vi "Expedite the Valley.vi"(0 "Valley in":T2[][](array[typedef]), 1 "Elf Locations in":set{T1}(c389)) -> (2 "Elf Locations out":set{T1}(c389), 3 "Valley out":T2[][](array[typedef]))   [LabVIEW 2020, in "AoC 2022.lvlib"]
uses:
  AoC 2022.lvlib
  Valley Point.ctl
  Valley Item.ctl
  Day 15 - Beacon Exclusion Zone/private/Location.ctl
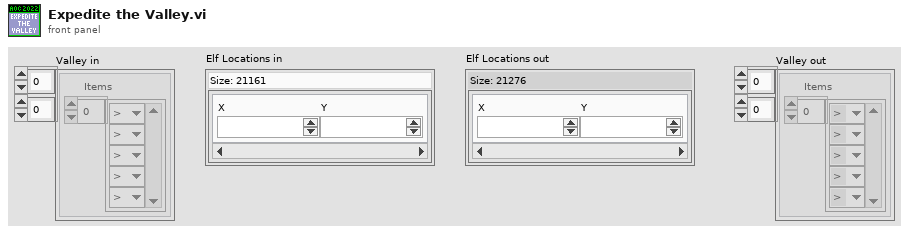
[diagram p1: front panel]
types:
  T1 = typedef "AoC 2022.lvlib/Location.ctl" = cluster{"X":i32, "Y":i32}
  T2 = typedef "AoC 2022.lvlib/Valley Point.ctl" = cluster{"Items":T3[]}
  T3 = typedef "AoC 2022.lvlib/Valley Item.ctl" = enum16{"#", ".", ">", "<", "^", "v", "E"}
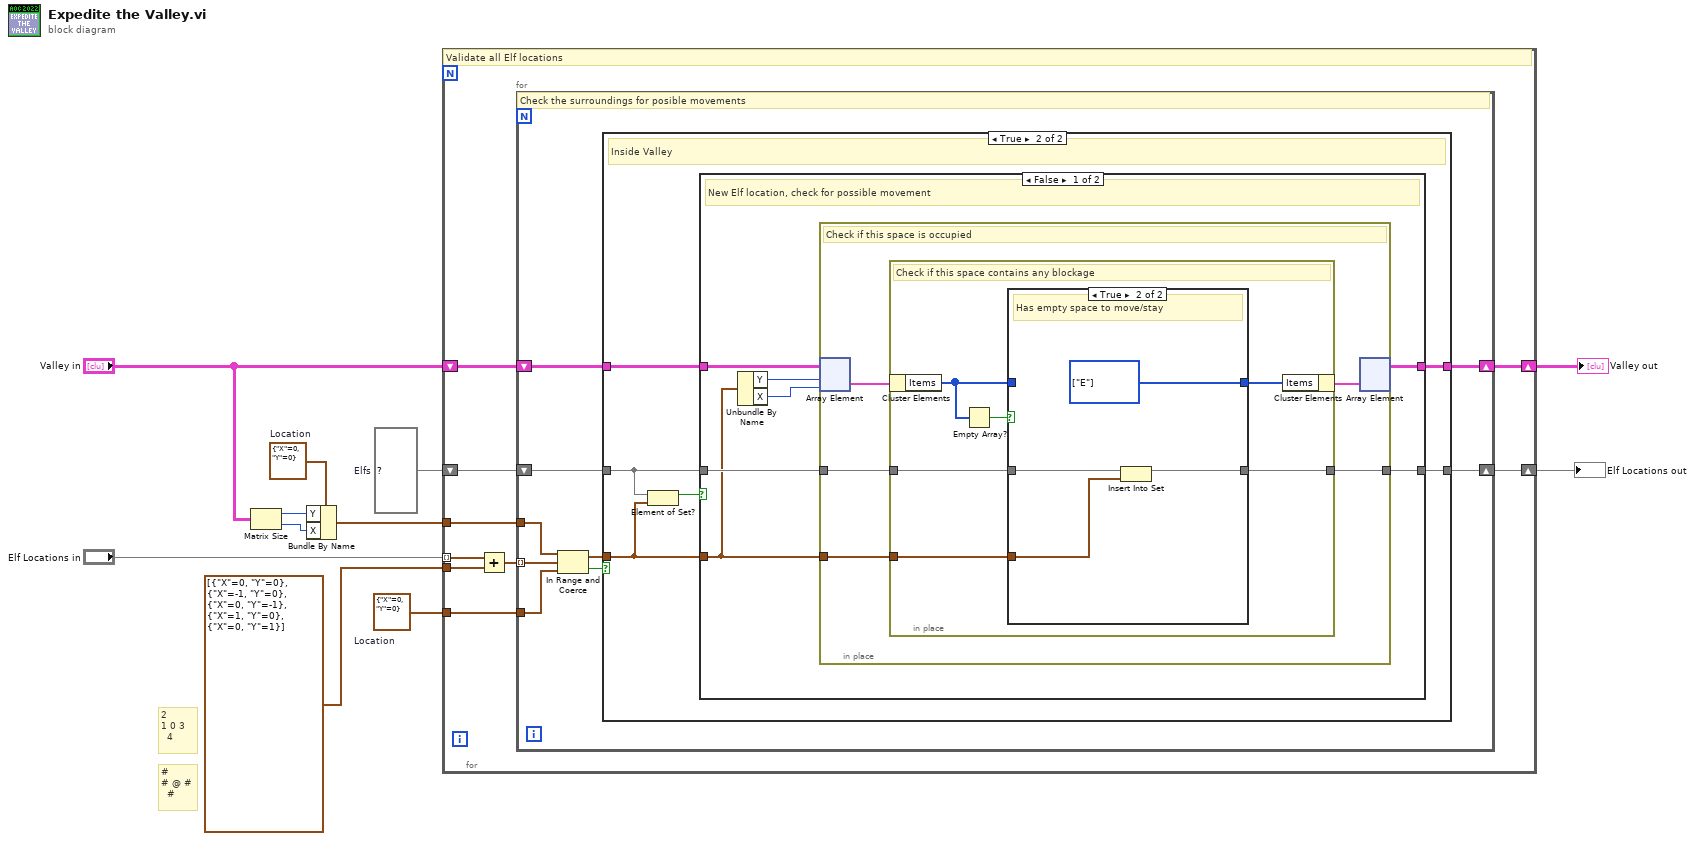
[diagram p0: block diagram]
diagram:
  w2 = set{T1} {}  # Elfs
  w3 = T1 {"X"=0, "Y"=0}  # Location
  w5 = T1 {"X"=0, "Y"=0}  # Location
  # "2  \n1 0 3\n  4"
  # "#  \n# @ #\n  #"
  n1 = Matrix Size(0:"Valley in") -> (1:w7:i32, 2:w6:i32)
  n2 = Bundle By Name(cluster=w5, "Y"=w7, "X"=w6) -> (w8:T1)
  n3 = for {
    shift-right: [w19] -> w11
    shift-left: "Valley in" -> [w20]
    tunnel: T1[] [{"X"=0, "Y"=0}, {"X"=-1, "Y"=0}, {"X"=0, "Y"=-1}, {"X"=1, "Y"=0}, {"X"=0, "Y"=1}] -> [w18]
    tunnel: w8 -> [w17]
    tunnel: "Elf Locations in" -> [w16] mode=indexing
    tunnel: w3 -> [w15]
    shift-right: [w12] -> w1
    shift-left: w2 -> [w13]
    # "Validate all Elf locations"
    n4 = Add(x=w16, y=w18) -> (x+y=w14:T1[])
    n5 = for {
      tunnel: w17 -> [w25]
      tunnel: w14 -> [w27] mode=indexing
      shift-right: [w28] -> w19
      shift-left: w20 -> [w29]
      tunnel: w15 -> [w26]
      shift-right: [w21] -> w12
      shift-left: w13 -> [w22]
      # "Check the surroundings for posible movements"
      n6 = In Range and Coerce(upper limit=w25, x=w27, lower limit=w26) -> (coerced(x)=w23:T1, In Range?=w24:bool)
      n7 = case shown="True" w24 {
        tunnel: w29 -> [w31 w37]
        tunnel: [w31 w36] -> w28
        tunnel: w23 -> [_ w33]
        tunnel: w22 -> [w30 w34]
        tunnel: [w30 w35] -> w21
        frame False {
          # "Outside Valley"
        }
        frame True {
          # "Inside Valley"
          n8 = Element of Set?(10:w33, 11:w34) -> (3:w32:bool)
          n9 = case shown="False" w32 {
            tunnel: w37 -> [w44 w63]
            tunnel: [w43 w63] -> w36
            tunnel: [w40 w62] -> w35
            tunnel: w34 -> [w39 w62]
            tunnel: w33 -> [w38 _]
            frame False {
              # "New Elf location, check for possible movement"
              n10 = Unbundle By Name(w38) -> ("Y"=w42:i32, "X"=w41:i32)
              n11 = in-place {
                in-place-border: w39 -> [w47]
                in-place-border: [w46] -> w40
                in-place-border: w38 -> [w45]
                # "Check if this space is occupied"
                n12 = in-place-array #1(w44, w42, w41) -> (w49:T2)
                n13 = in-place {
                  in-place-border: w47 -> [w54]
                  in-place-border: [w53] -> w46
                  in-place-border: w45 -> [w50]
                  # "Check if this space contains any blockage"
                  n14 = in-place-cluster #2(w49) -> ("Items"=w52:T3[])
                  n15 = Empty Array?(array=w52) -> (empty?=w51:bool)
                  n16 = case shown="True" w51 {
                    tunnel: [w56 w61] -> w55
                    tunnel: w54 -> [w57 w60]
                    tunnel: [w57 w59] -> w53
                    tunnel: w52 -> [w56 _]
                    tunnel: w50 -> [_ w58]
                    frame False {
                      # "Blocked"
                    }
                    frame True {
                      w61 = T3[] [enum."E"] items=["#", ".", ">", "<", "^", "v", "E"]
                      # "Has empty space to move/stay"
                      n17 = Insert Into Set(10:w58, 11:w60) -> (3:w59:set{T1})  [unwired: 1 out]
                    }
                  }
                  n18 = in-place-cluster #2("Items"=w55) -> (w48:T2)
                }
                n19 = in-place-array #1(w48) -> (w43:T2[][])  [unwired: 2 out]
              }
            }
            frame True {
              # "Elf location already added"
            }
          }
        }
      }
    }
  }
  "Valley out" <- w11
  "Elf Locations out" <- w1
